vi "ChangeAmpCh1.vi"(0 "object in":refnum<class "AFG3022B_OJ.lvclass">, 2 "Amplitude (1 Vpp)":dbl, 5 "error in (no error)":errorcluster) -> (14 "object out":refnum<class "AFG3022B_OJ.lvclass">, 19 "error out":errorcluster)   [LabVIEW 2023, in "AFG3022B_OJ.lvclass"]
uses:
  AFG3022B_OJ.lvclass
  AFG3022B_OJ.lvclass/AFG3022B_OJ.ctl
  <instrlib>/Tektronix AFG 3000 Series/Tektronix AFG 3000 Series.lvlib
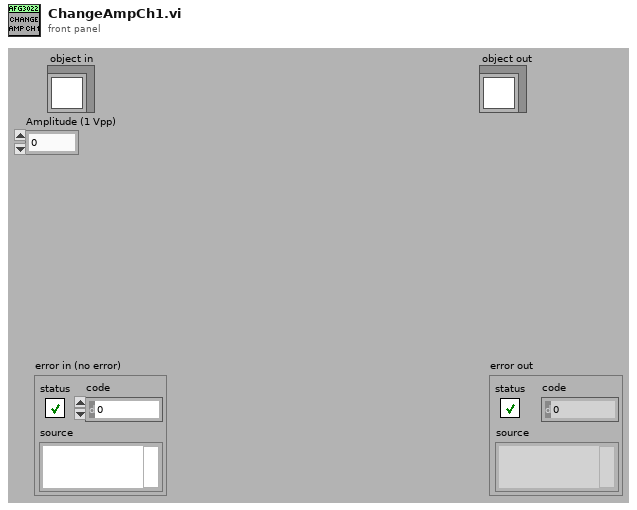
[diagram p1: front panel]
types:
  T1 = cluster{"Frequency Hz (1000 Hz)":dbl, "Waveform Function (0: Sine)":u16, "Amplitude (1 Vpp)":dbl, "DC Offset (0.00 V)":dbl, "Phase Level (-1)":dbl, "Phase Unit (0: Radian)":u16}
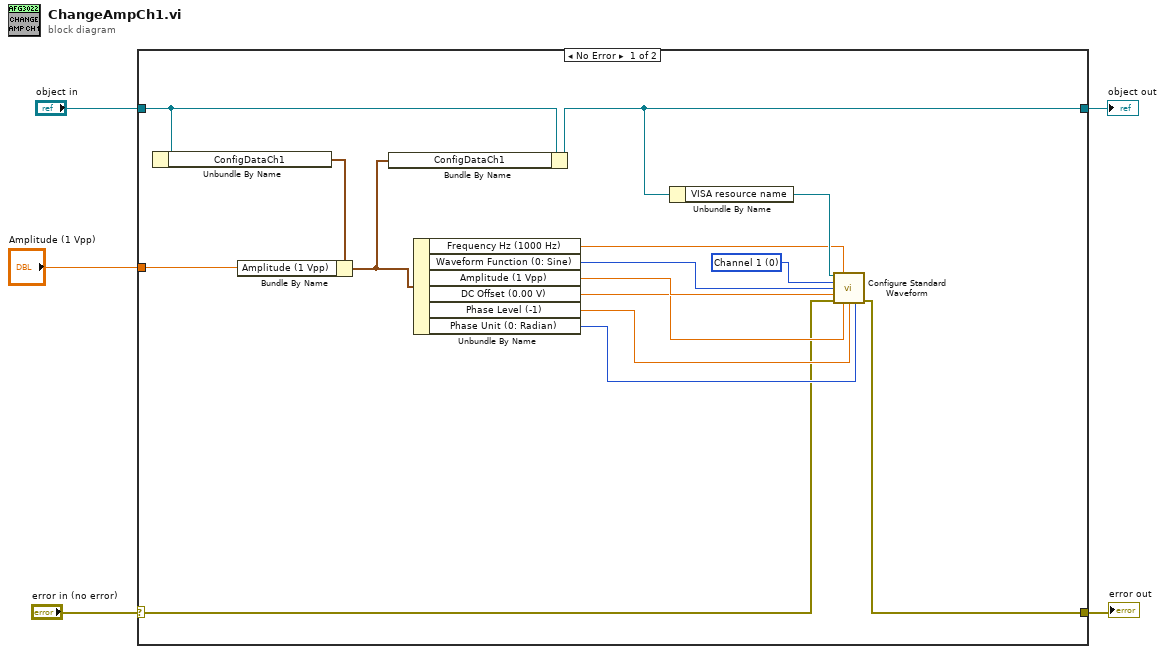
[diagram p0: block diagram]
diagram:
  n1 = case shown="No Error" "error in (no error)" {
    selector: "error in (no error)" -> [w8 w22]
    tunnel: [w7 w22] -> w4
    tunnel: [w12 w21] -> w2
    tunnel: "object in" -> [w11 w21]
    tunnel: "Amplitude (1 Vpp)" -> [w6 _]
    frame No Error {
      w13 = u16 0 items=["Channel 1", "Channel 2"] ("Channel (0: Channel 1)")
      n2 = Unbundle By Name(w11) -> ("ConfigDataCh1"=w10:T1)
      n3 = Bundle By Name(cluster=w10, "Amplitude (1 Vpp)"=w6) -> (w9:T1)
      n4 = Bundle By Name(cluster=w11, "ConfigDataCh1"=w9) -> (w12:refnum<class "AFG3022B_OJ.lvclass">)
      n5 = Unbundle By Name(w9) -> ("Frequency Hz (1000 Hz)"=w19:dbl, "Waveform Function (0: Sine)"=w18:u16, "Amplitude (1 Vpp)"=w17:dbl, "DC Offset (0.00 V)"=w16:dbl, "Phase Level (-1)"=w15:dbl, "Phase Unit (0: Radian)"=w14:u16)
      n6 = Unbundle By Name(w12) -> ("VISA resource name"=w20:refnum<visa-resource-name>)
      n7 = call <instrlib>:"Configure Standard Waveform.vi"("VISA resource name"=w20, "Frequency (1000 Hz)"=w19, "Channel (0: Channel 1)"=w13, "Waveform Function (0: Sine)"=w18, "Amplitude (1 Vpp)"=w17, "error in (no error)"=w8, "DC Offset (0.00 V)"=w16, "Phase Level (-1)"=w15, "Phase Unit (0: Radian)"=w14) -> ("error out"=w7:errorcluster)  [unwired: 5 in, 1 out]
    }
    frame Error {
    }
  }
  "error out" <- w4
  "object out" <- w2
